vi "2_Hot_Films_13_1_00.vi"() -> (5 "Plug in titles":string[](array[string]), 7 "Plug in values":string[](array[string]))   [LabVIEW 2010]
uses:
  Controls/Post_Process.ctl
  Globals/Meas_global.vi
  Globals/Plug_in_data_global.vi
  <vilib>/Analysis/3filter.llb/Butterworth Filter (DBL).vi
  <vilib>/Analysis/NI_AALBase.lvlib
  <vilib>/Analysis/NI_AALPro.lvlib
panel:
  in  "Case Constant\n(See Context Help)":bool
  out "Array":string[](array[string])
  out "Max Correlation":dbl format="%.2f"
  in  "Approx Delay (s)":dbl=23.0 format="%.2f"
  out "XY Graph":cluster{dbl[], dbl[]}[](graph)
  out "Hot Film mean":dbl format="%.2f"
  out "ADV mean":dbl format="%.2f"
  in  "Approx period":dbl=80.0 format="%.2f"
  in  "Block Length":i32=200
  in  "Start chop":i32=2000
  out "Trailing Auto correlation":cluster{dbl, dbl, dbl[]}[](graph)
  out "U components":cluster{dbl[], dbl[]}[](graph)
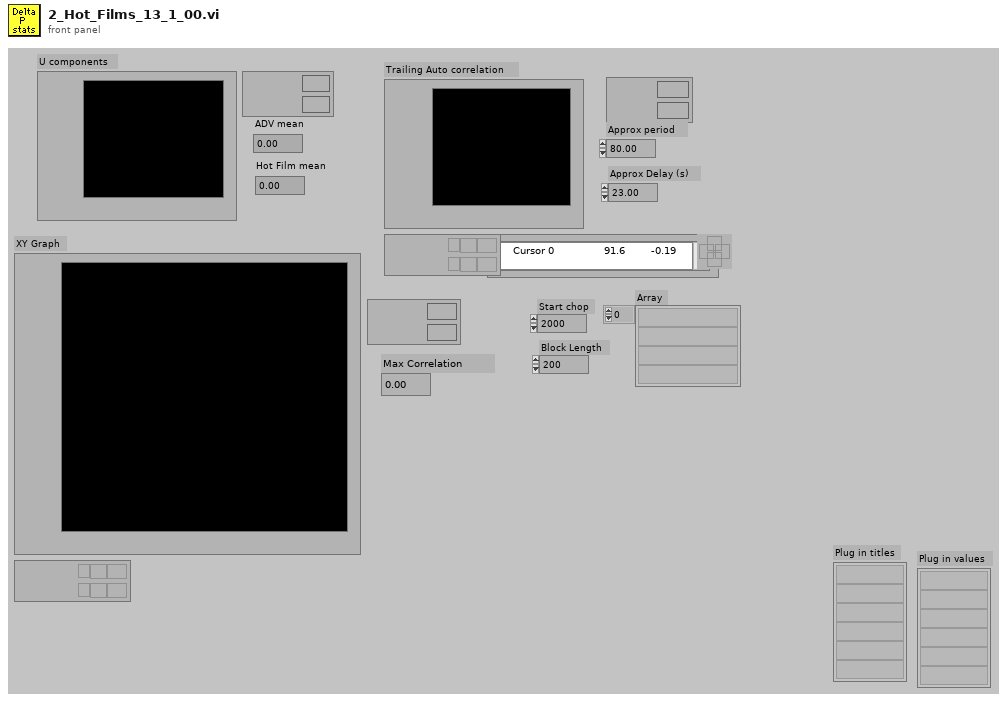
[diagram p1: front panel]
types:
  T1 = enum32{"Lowpass", "Highpass", "Bandpass", "Bandstop"}
  T2 = typedef "Post_Process.ctl" = enum16{"Take New Data", "Post Process Raw Data File"}
  T3 = cluster{"X array Out":dbl[], "Y array Out":dbl[]}
  T4 = cluster{"X array Out":dbl[], "Y array Out":dbl[]}[]
  T5 = typedef "Analysis_info_cluster.ctl" = cluster{"Colour":u32, "Inst type":T6, "Inst name":string, "Symbol":string, "Code name":string, "Extra Info":string, "Inst Array":T7, "Index":i32, "Voltage Index":i32, "Extra Titles":string[], "Extra Values":string[]}
  T6 = typedef "Inst_type.ctl" = enum16{"Propeller anemometer", "Raw voltage", "Pressure Transducer", "Pitot-static tube", "Preston tube", "Hot wire", "Cross wire 1", "Cross wire 2", "Generic Linear", "Generic Polynomial", "Generic BackPoly", "Fast FID", "Thermocouple", "Cold wire", "Pulsed Wire", "LDA Vel", "LDA Tran time", "LDA Arr time"}
  T7 = typedef "Instrument_Array.ctl" = enum16{"PWA", "LDA", "Analogue"}
  T8 = cluster{"Name":string, "X":dbl, "Y":dbl, "Z":dbl}[]
  T9 = cluster{"Name":string, "X":dbl, "Y":dbl, "Z":dbl}
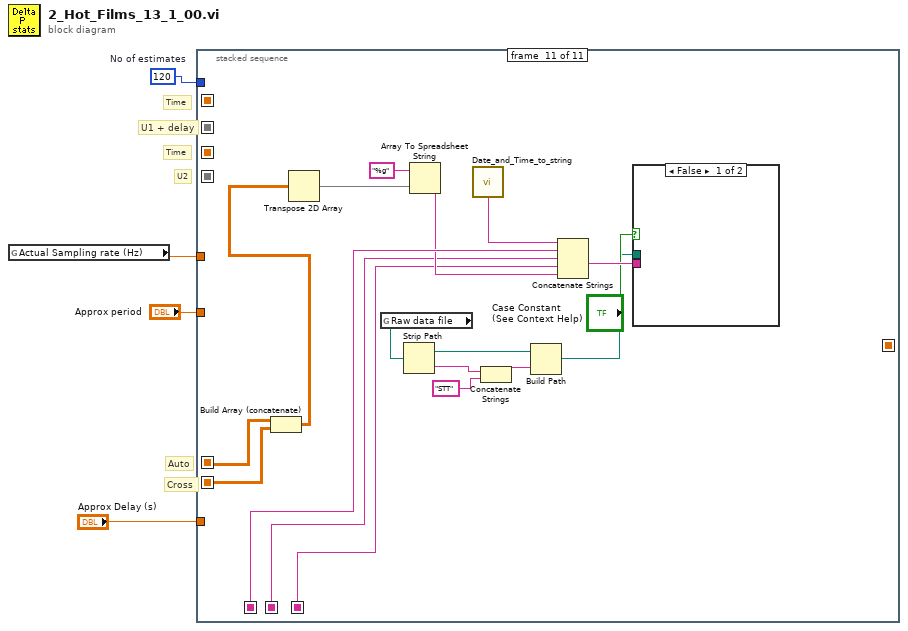
[diagram p0: block diagram]
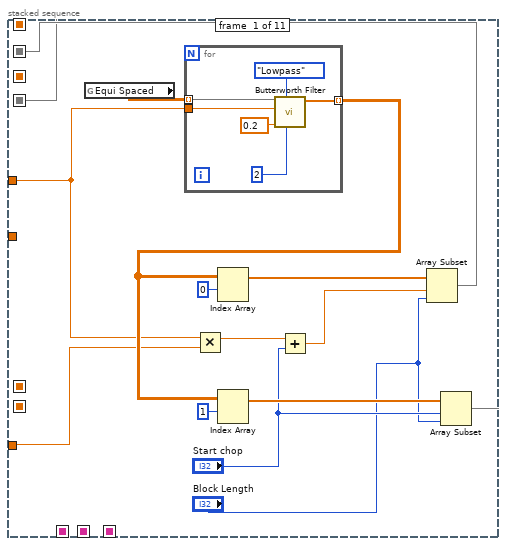
[diagram p2: hidden frame]
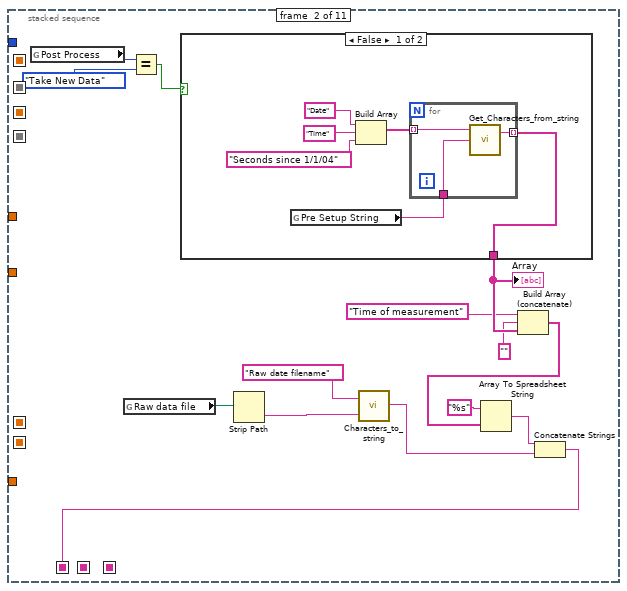
[diagram p3: hidden frame]
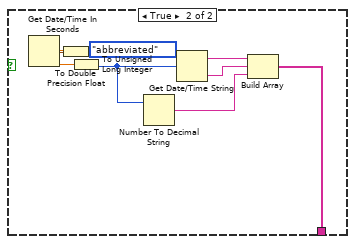
[diagram p4: hidden frame]
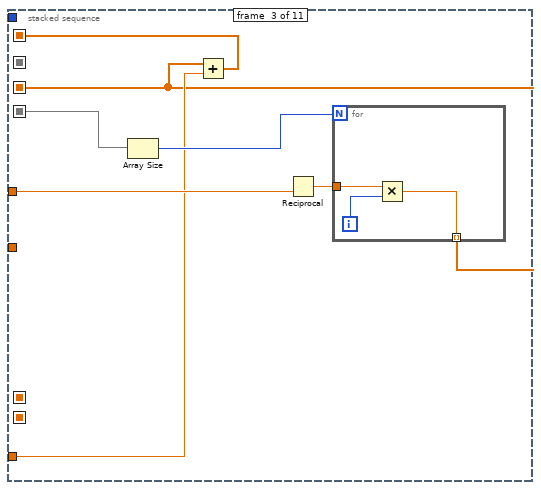
[diagram p5: hidden frame]
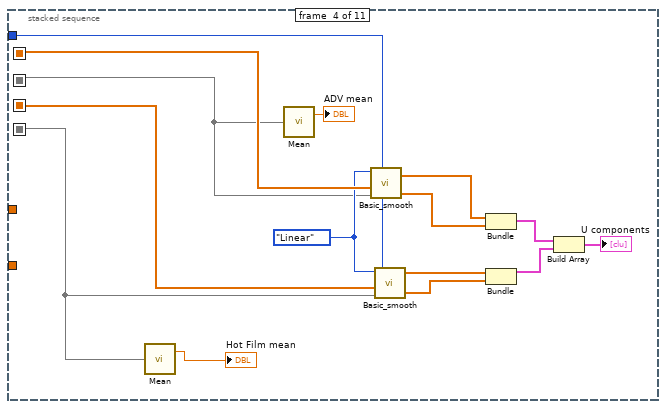
[diagram p6: hidden frame]
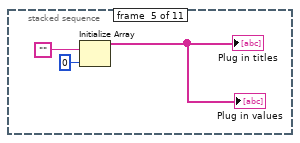
[diagram p7: hidden frame]
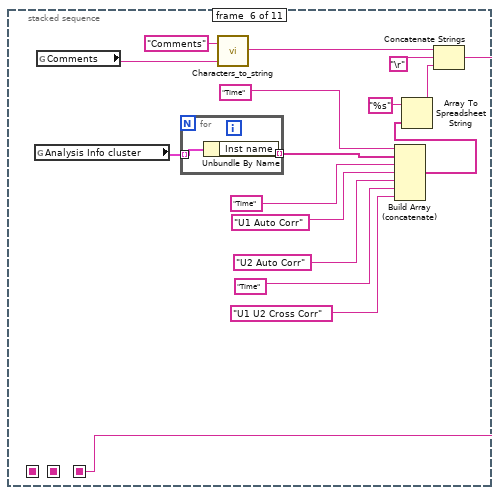
[diagram p8: hidden frame]
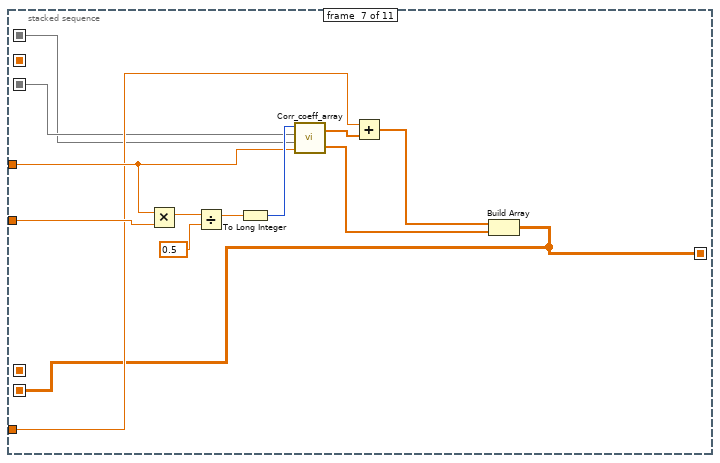
[diagram p9: hidden frame]
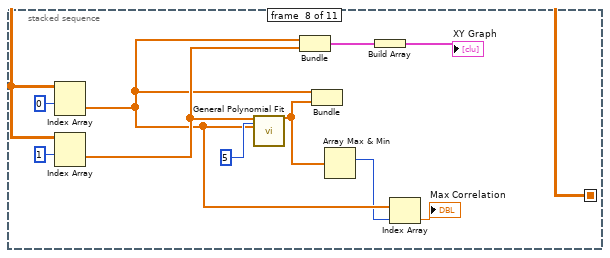
[diagram p10: hidden frame]
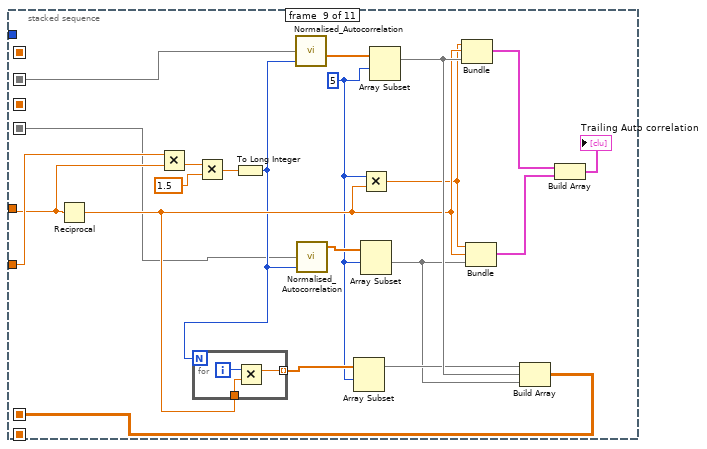
[diagram p11: hidden frame]
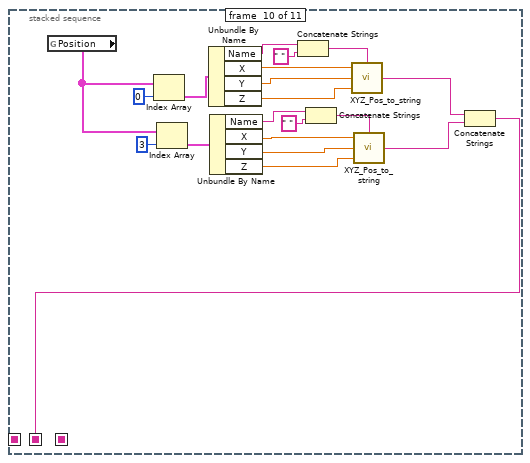
[diagram p12: hidden frame]
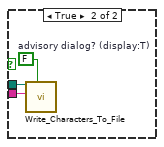
[diagram p13: hidden frame]
diagram:
  w4 = 120  # No of estimates
  # "Time"
  # "Time"
  # "U2"
  # "U1 + delay"
  # "Cross"
  # "Auto"
  n1 = global read "Meas_global.vi" "Actual Sampling rate (Hz)"() -> (w2:dbl)
  n2 = stacked-sequence {
    seq-local: [_ _ _ _ _ w95 _ _ _ _ _] -> [_ _ _ _ _ _ _ _ _ _ w177]
    seq-local: [_ w31 _ _ _ _ _ _ _ _ _] -> [_ _ _ _ _ _ _ _ _ _ w186]
    seq-local: [_ _ _ _ _ _ _ _ w146 _ _] -> [_ _ _ _ _ _ _ _ _ _ w182]
    seq-local: [_ _ _ _ _ _ w104 _ _ _ _] -> [_ _ _ _ _ _ _ _ _ _ w181]
    seq-local: [_ _ _ _ _ _ _ _ _ w155 _] -> [_ _ _ _ _ _ _ _ _ _ w176]
    seq-local: [_ _ _ _ _ _ w104 _ _ _ _] -> [_ _ _ _ _ _ _ w123 _ _ _]
    seq-local: [w9 _ _ _ _ _ _ _ _ _ _] -> [_ _ _ w67 _ _ w102 _ w127 _ _]
    seq-local: [w8 _ _ _ _ _ _ _ _ _ _] -> [_ _ w60 w66 _ _ w103 _ w126 _ _]
    seq-local: [_ _ w56 _ _ _ _ _ _ _ _] -> [_ _ _ w76 _ _ _ _ _ _ _]
    seq-local: [_ _ w57 _ _ _ _ _ _ _ _] -> [_ _ _ w72 _ _ _ _ _ _ _]
    tunnel: w2 -> [w12 _ w61 _ _ _ w111 _ w144 _ _]
    tunnel: w4 -> [_ _ _ w69 _ _ _ _ _ _ _]
    tunnel: "Approx period" -> [_ _ _ _ _ _ w114 _ w145 _ _]
    tunnel: "Approx Delay (s)" -> [w13 _ w58 _ _ _ w106 _ _ _ _]
    frame #0 {
      n3 = global read "Plug_in_data_global.vi" "Equi Spaced"() -> (w18:dbl[][])
      n4 = for {
        tunnel: [w21] -> w15 mode=indexing
        tunnel: w12 -> [w20]
        tunnel: w18 -> [w19] mode=indexing
        n5 = call-poly <vilib>:"Butterworth Filter.vi"("order"=2, "filter type"=T1."Lowpass", "low cutoff freq: fl"=0.2, "sampling freq: fs"=w20, "X"=w19) -> ("Filtered X"=w21:dbl[])  [unwired: 3 in, 1 out]
      }
      n6 = Multiply(x=w12, y=w13) -> (x*y=w11:dbl)
      n7 = Index Array(array=w15, index (row)=0 ("Index")) -> (element=w14:dbl[])  [unwired: 1 in]
      n8 = Index Array(array=w15, index (row)=1 ("Index")) -> (element=w7:dbl[])  [unwired: 1 in]
      n9 = Add(x=w11, y="Start chop") -> (x+y=w10:dbl)
      n10 = Array Subset(array=w14, index=w10, length="Block Length") -> (w9:dbl[])
      n11 = Array Subset(array=w7, index="Start chop", length="Block Length") -> (w8:dbl[])
    }
    frame #1 {
      n12 = global read "Meas_global.vi" "Post Process"() -> (w37:T2)
      n13 = global read "Meas_global.vi" "Raw data file"() -> (w26:path)
      n14 = Equal?(x=w37, y=Post_Process."Take New Data" ("Post Process")) -> (x = y?=w36:bool)
      n15 = case shown="False" w36 {
        tunnel: [w39 w49] -> w30
        frame False {
          n16 = global read "Meas_global.vi" "Pre Setup String"() -> (w40:string)
          n17 = Build Array("Date", "Time", "Seconds since 1/1/04") -> (w41:string[])
          n18 = for {
            tunnel: w41 -> [w47] mode=indexing
            tunnel: w40 -> [w46]
            tunnel: [w45] -> w39 mode=indexing
            n19 = call "Get_Characters_from_string.vi"("Input string"=w46, "Variable name"=w47) -> ("Value"=w45:string)  [unwired: 1 in, 1 out]
          }
        }
        frame True {
          n20 = Get Date/Time In Seconds() -> (seconds since 1Jan1904=w48:timestamp)
          n21 = To Double Precision Float(number=w48) -> (double precision float=w52:dbl)
          n22 = To Unsigned Long Integer(number=w52) -> (unsigned 32bit integer=w51:u32)
          n23 = Number To Decimal String(number=w51) -> (decimal integer string=w50:string)  [unwired: 1 in]
          n24 = Get Date/Time String(date format (0)=enum16{"short", "long", "abbreviated"}."abbreviated", seconds (now)=w51) -> (date string=w54:string, time string=w53:string)  [unwired: 1 in]
          n25 = Build Array(w54, w53, w50) -> (w49:string[])
        }
      }
      "Array" <- w30
      n26 = Strip Path(path=w26) -> (name=w25:string)  [unwired: 1 out]
      n27 = call "Characters_to_string.vi"("Characters to write"=w25, "Label for characters"="Raw date filename") -> ("Output string"=w32:string)
      n28 = Build Array (concatenate)("Time of measurement", "" ("Value"), w30) -> (w27:string[])
      n29 = Array To Spreadsheet String(array=w27, 3:"%s" ("format string")) -> (spreadsheet string=w33:string)  [unwired: 1 in]
      n30 = Concatenate Strings(w33, w32) -> (w31:string)
    }
    frame #2 {
      n31 = Array Size(array=w60) -> (size(s)=w59:i32)
      n32 = Reciprocal(x=w61) -> (1/x=w62:dbl)
      n33 = for {
        N: w59 -> [_]
        tunnel: w62 -> [w65]
        tunnel: [w63] -> w57 mode=indexing
        i -> [w64]
        n34 = Multiply(x=w65, y=w64) -> (x*y=w63:dbl)
      }
      n35 = Add(x=w57, y=w58) -> (x+y=w56:dbl[])
    }
    frame #3 {
      w73 = enum16{"Linear", "Logarithmic"}."Linear" ("Smoothing")
      n36 = call <vilib>:"Mean.vi"("X"=w66) -> ("mean"=→"Hot Film mean":dbl)  [unwired: 1 out]
      n37 = call <vilib>:"Mean.vi"("X"=w67) -> ("mean"=→"ADV mean":dbl)  [unwired: 1 out]
      n38 = call "Basic_smooth.vi"("Smoothing"=w73, "X array in"=w76, "Y array in"=w67, "No of estimates output"=w69) -> ("X array Out"=w75:dbl[], "Y array Out"=w74:dbl[])  [unwired: 1 in]
      n39 = call "Basic_smooth.vi"("Smoothing"=w73, "X array in"=w72, "Y array in"=w66, "No of estimates output"=w69) -> ("X array Out"=w71:dbl[], "Y array Out"=w70:dbl[])  [unwired: 1 in]
      n40 = Bundle("X array Out"=w75, "Y array Out"=w74) -> (w80:T3)  [unwired: 1 in]
      n41 = Bundle("X array Out"=w71, "Y array Out"=w70) -> (w79:T3)  [unwired: 1 in]
      n42 = Build Array(w80, w79) -> (→"U components":T4)
    }
    frame #4 {
      n43 = Initialize Array("", 0) -> (→"Plug in titles" →"Plug in values":string[])
    }
    frame #5 {
      n44 = global read "Meas_global.vi" "Analysis Info cluster"() -> (w94:T5[])
      n45 = global read "Meas_global.vi" "Comments"() -> (w99:string)
      n46 = for {
        tunnel: w94 -> [w101] mode=indexing
        tunnel: [w100] -> w87 mode=indexing
        n47 = Unbundle By Name(w101) -> ("Inst name"=w100:string)
      }
      n48 = call "Characters_to_string.vi"("Characters to write"=w99, "Label for characters"="Comments") -> ("Output string"=w97:string)
      n49 = Build Array (concatenate)("Time", w87, "Time", "U1 Auto Corr", "U2 Auto Corr", "Time", "U1 U2 Cross Corr") -> (w90:string[])
      n50 = Array To Spreadsheet String(array=w90, 3:"%s" ("format string")) -> (spreadsheet string=w89:string)  [unwired: 1 in]
      n51 = Concatenate Strings(w97, "\r", w89) -> (w95:string)
    }
    frame #6 {
      n52 = Multiply(x=w111, y=w114) -> (x*y=w110:dbl)
      n53 = Divide(x=w110, y=0.5) -> (x/y=w108:dbl)
      n54 = To Long Integer(number=w108) -> (32bit integer=w113:i32)
      n55 = call "Corr_coeff_array.vi"("Sampling frequency"=w111, "U2"=w102, "U1"=w103, "Slippage range"=w113) -> ("Correlation Coefficient"=w112:dbl[], "Time"=w107:dbl[])
      n56 = Add(x=w106, y=w107) -> (x+y=w105:dbl[])
      n57 = Build Array(w105, w112) -> (w104:dbl[][])
    }
    frame #7 {
      n58 = Index Array(array=w123, index (row)=0 ("Index")) -> (element=w117:dbl[])  [unwired: 1 in]
      n59 = Index Array(array=w123, index (row)=1 ("Index")) -> (element=w120:dbl[])  [unwired: 1 in]
      n60 = call <vilib>:"General Polynomial Fit.vi"("Y"=w120, "polynomial order"=5, "X"=w117) -> ("Best Polynomial Fit"=w118:dbl[])  [unwired: 9 in, 3 out]
      n61 = Bundle(w117, w120) -> (w122:cluster{dbl[], dbl[]})  [unwired: 1 in]
      n62 = Bundle(w117, "Best Polynomial Fit"=w118) -> ()  [unwired: 1 in, 1 out]
      n63 = Array Max & Min(array=w118) -> (max index (indices)=w116:i32)  [unwired: 3 out]
      n64 = Build Array(w122) -> (→"XY Graph":cluster{dbl[], dbl[]}[])
      n65 = Index Array(array=w117, index=w116) -> (element=→"Max Correlation":dbl)
    }
    frame #8 {
      w133 = 5
      n66 = Reciprocal(x=w144) -> (1/x=w135:dbl)
      n67 = Multiply(x=w145, y=w144) -> (x*y=w143:dbl)
      n68 = Multiply(x=w143, y=1.5) -> (x*y=w141:dbl)
      n69 = To Long Integer(number=w141) -> (32bit integer=w132:i32)
      n70 = for {
        N: w132 -> [_]
        tunnel: w135 -> [w148]
        tunnel: [w147] -> w137 mode=indexing
        i -> [w149]
        n71 = Multiply(x=w149, y=w148) -> (x*y=w147:dbl)
      }
      n72 = call "Normalised_Autocorrelation.vi"("Autocorrelation length"=w132, "Array"=w127) -> ("Normalised Auto corr"=w140:dbl[])  [unwired: 1 in]
      n73 = call "Normalised_Autocorrelation.vi"("Autocorrelation length"=w132, "Array"=w126) -> ("Normalised Auto corr"=w139:dbl[])  [unwired: 1 in]
      n74 = Array Subset(array=w137, index=w133) -> (w136:dbl[])  [unwired: 1 in]
      n75 = Multiply(x=w133, y=w135) -> (x*y=w134:dbl)
      n76 = Array Subset(array=w139, index=w133) -> (w131:dbl[])  [unwired: 1 in]
      n77 = Array Subset(array=w140, index=w133) -> (w138:dbl[])  [unwired: 1 in]
      n78 = Bundle(w134, w135, w138) -> (w129:cluster{dbl, dbl, dbl[]})  [unwired: 1 in]
      n79 = Bundle(w134, w135, w131) -> (w130:cluster{dbl, dbl, dbl[]})  [unwired: 1 in]
      n80 = Build Array(w136, w138, w131) -> (w146:dbl[][])
      n81 = Build Array(w129, w130) -> (→"Trailing Auto correlation":cluster{dbl, dbl, dbl[]}[])
    }
    frame #9 {
      n82 = global read "Meas_global.vi" "Position"() -> (w167:T8)
      n83 = Index Array(array=w167, index=0) -> (element=w166:T9)
      n84 = Index Array(array=w167, index=3) -> (element=w165:T9)
      n85 = Unbundle By Name(w166) -> ("Name"=w152:string, "X"=w163:dbl, "Y"=w162:dbl, "Z"=w161:dbl)
      n86 = Unbundle By Name(w165) -> ("Name"=w150:string, "X"=w160:dbl, "Y"=w159:dbl, "Z"=w158:dbl)
      n87 = Concatenate Strings(w152, " " ("Output string")) -> (w164:string)
      n88 = Concatenate Strings(w150, " " ("Output string")) -> (w154:string)
      n89 = call "XYZ_Pos_to_string.vi"("Position label"=w164, "Z"=w161, "Y"=w162, "X"=w163) -> ("Output string"=w157:string)
      n90 = call "XYZ_Pos_to_string.vi"("Position label"=w154, "Z"=w158, "Y"=w159, "X"=w160) -> ("Output string"=w156:string)
      n91 = Concatenate Strings(w157, w156) -> (w155:string)
    }
    frame #10 {
      n92 = Build Array (concatenate)(w182, w181) -> (w179:dbl[][])
      n93 = Transpose 2D Array(2D array=w179) -> (transposed array=w187:dbl[][])
      n94 = global read "Meas_global.vi" "Raw data file"() -> (w174:path)
      n95 = Strip Path(path=w174) -> (stripped path=w171:path, name=w173:string)
      n96 = Array To Spreadsheet String(array=w187, 3:"%g" ("format string")) -> (spreadsheet string=w178:string)  [unwired: 1 in]
      n97 = call "Date_and_Time_to_string.vi"() -> ("Date and time (spreadsheet)"=w180:string)
      n98 = Concatenate Strings(w173, "STT") -> (w172:string)
      n99 = Build Path(base path=w171, name or relative path=w172) -> (appended path=w170:path)
      n100 = Concatenate Strings(w180, w186, w176, w177, w178) -> (w184:string)
      n101 = case shown="False" "Case Constant\n(See Context Help)" {
        tunnel: w184 -> [_ w190]
        tunnel: w170 -> [_ w189]
        frame False {
        }
        frame True {
          w188 = FALSE  # advisory dialog? (display:T)
          n102 = call "Write_Characters_To_File.vi"("file path (dialog if empty)"=w189, "advisory dialog? (display:T)"=w188, "character string"=w190) -> ()  [unwired: 5 in, 1 out]
        }
      }
    }
  }
